vi "Quick Start - Simple - Write Data.vi"() -> ()   [LabVIEW 2020]
uses:
  Nominal Client/Nominal Client.lvclass/Nominal Client.ctl
  8bc873d6-11f2-47b8-afa9-2ee06eb45ce7.vi
  44f76e3e-3723-4288-9350-5dd63fde3615.vi
  4190ffb6-c6fc-4755-9f25-b1780647bb6c.vi
  Nominal Client/private_data.set.vi
  4190ffb6-c6fc-4755-9f25-b1780647bb6c.vi/028fdd67-09da-40c6-8995-0c4bd62a0b31.vi
  <vilib>/JDP Science/JSONtext/Make JSON Object.vi
  4190ffb6-c6fc-4755-9f25-b1780647bb6c.vi/c2a1aca9-ea5a-4b2a-8072-18de54756c53.vi
  <vilib>/JDP Science/JSONtext/Make JSON Array.vi
  4190ffb6-c6fc-4755-9f25-b1780647bb6c.vi/2c8a2fb0-06af-4bda-9dcc-d72a85547e70.vi
  <vilib>/LabVIEW Open Source Project/Epoch Date & Time/epoch.UNIX/Epoch.UNIX.lvclass
  C:/Program Files/National Instruments/LabVIEW 2020/vi.lib/LabVIEW Open Source Project/Epoch Date & Time/epoch/Epoch.lvclass
  <vilib>/Utility/file.llb/Application Directory.vi
  <vilib>/Utility/error.llb/Error Cluster From Error Code.vi
  submodules/reqwest-labview/lv-src/reqwest/create.vi
  <vilib>/LabVIEW Open Source Project/Epoch Date & Time/Get Epoch Time.vi
  nominal types/properties/create.from_map.vi
  Nominal Client/nominal_channel_writer.write_batches.path.vi
  <vilib>/JDP Science/JSONtext/Variant to JSON Text.vi
  <vilib>/JDP Science/JSONtext/support/Format JSON Object.vi
  <vilib>/JDP Science/JSONtext/support/Format JSON Array Text.vi
  Nominal Client/http.post.vi
  Nominal Client/Nominal Client.lvclass
  nominal types/workspace/workspace.lvclass
  submodules/reqwest-labview/lv-src/reqwest/reqwest.lvclass
  <vilib>/JDP Science/JSONtext/LVClass Serializer/JSONtext LVClass Serializer.lvclass
  nominal types/properties/properties.lvclass
panel:
  in  "Data Source RID":string
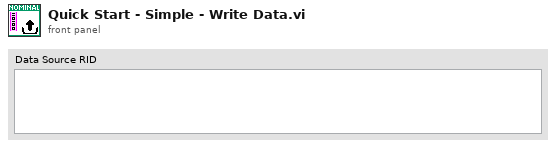
[diagram p1: front panel]
types:
  T1 = cluster{"UNIX Timestamp":cluster{"Seconds":i64, "Nanoseconds":i64}, "number: 0 to 1":dbl}
  T2 = cluster{"Channel":string, cluster{"UNIX Timestamp":cluster{"Seconds":i64, "Nanoseconds":i64}, "number: 0 to 1":dbl}[]}
  T3 = cluster{"Channel":string, cluster{"UNIX Timestamp":cluster{"Seconds":i64, "Nanoseconds":i64}, "number: 0 to 1":dbl}[]}[]
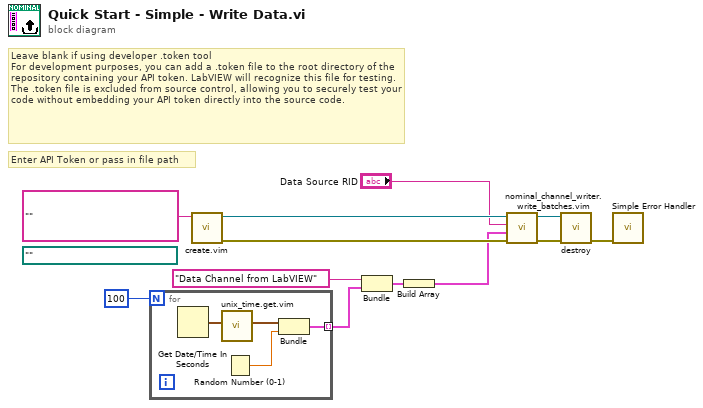
[diagram p0: block diagram]
diagram:
  (unwired) path ""
  # "Leave blank if using developer .token tool\nFor development purposes, you can add a .token file to the root directory of the repository containing your API token. LabVIEW will recognize this file for testing. The .token file is excluded from source control, allowing you to securely test your code without embedding your API token directly into the source code."
  # "Enter API Token or pass in file path"
  n1 = for {
    N: 100 -> [_]
    tunnel: [w13] -> w5 mode=indexing
    n2 = Get Date/Time In Seconds() -> (seconds since 1Jan1904=w16:timestamp)
    n3 = call "unix_time.get.vim"("Time Stamp (empty: now) [single or array]"=w16) -> ("UNIX Timestamp"=w15:cluster{"Seconds":i64, "Nanoseconds":i64})  [unwired: 10 in]
    n4 = Random Number (0-1)() -> (number: 0 to 1=w14:dbl)
    n5 = Bundle("UNIX Timestamp"=w15, "number: 0 to 1"=w14) -> (w13:T1)  [unwired: 1 in]
  }
  n6 = call "create.vim"("API Token (string or path)"="" ("API Token")) -> ("error out"=w11:errorcluster, "Nominal Client"=w12:refnum<class "Nominal Client.lvclass">)  [unwired: 9 in]
  n7 = Bundle("Channel"="Data Channel from LabVIEW", w5) -> (w4:T2)  [unwired: 1 in]
  n8 = Build Array(w4) -> (w1:T3)
  n9 = call "nominal_channel_writer.write_batches.vim"("error in"=w11, "batches"=w1, "Data Source RID"="Data Source RID", "Nominal Client in"=w12) -> ("error out"=w8:errorcluster, "Nominal Client out"=w9:refnum<class "Nominal Client.lvclass">)  [unwired: 5 in, 1 out]
  n10 = call "destroy.vi"("error in"=w8, "Nominal Client"=w9) -> ("error out"=w10:errorcluster)  [unwired: 9 in]
  n11 = call <vilib>:"Simple Error Handler.vi"("error in (no error)"=w10) -> ()  [unwired: 4 in, 5 out]
